vi "Server Base URL.vi"(11 "API Server (auto)":T1) -> (3 "Server Base URI":string)   [LabVIEW 2020, in "GCentral-API.lvlib"]
uses:
  GCentral-API.lvlib
  API Server.ctl
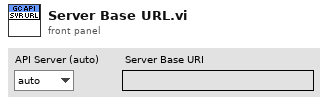
[diagram p1: front panel]
types:
  T1 = typedef "GCentral-API.lvlib/API Server.ctl" = enum16{"auto", "live", "test", "local"}
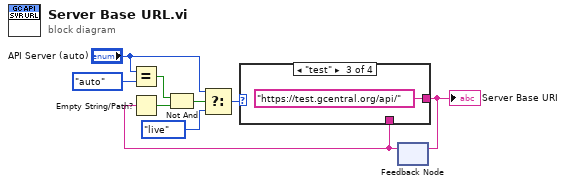
[diagram p0: block diagram]
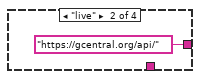
[diagram p3: hidden frame]
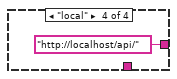
[diagram p4: hidden frame]
diagram:
  n1 = Equal?(x="API Server (auto)", y=API_Server."auto") -> (x = y?=w6:bool)
  n2 = feedback #1() -> (w7:string)  [unwired: 1 in]
  n3 = Empty String/Path?(string/path=w7) -> (empty?=w5:bool)
  n4 = Not And(1:w5, 2:w6) -> (0:w4:bool)
  n5 = Select(t="API Server (auto)", s=w4, f=API_Server."live" ("y")) -> (s? t:f=w1:T1)
  n6 = case shown="\"test\"" w1 {
    tunnel: [w10 "https://gcentral.org/api/" "https://test.gcentral.org/api/" "http://localhost/api/"] -> w9
    tunnel: w7 -> [w10 _ _ _]
    frame "auto" {
    }
    frame "live" {
    }
    frame "test" {
    }
    frame "local" {
    }
  }
  "Server Base URI" <- w9
  n7 = feedback-in #1(w9) -> ()
